vi "Documentation.vi"   [LabVIEW 2019, in "Inst.Transport.lvclass"]
uses:
  Inst.Transport.lvclass
  Typedefs/Inst.Transport.getAll--Cluster.ctl
  Typedefs/Inst.Transport.Configuration--Cluster.ctl
  <userlib>/LevyLab/Instrument Framework/Instrument/Instrument.lvclass
  <vilib>/JKI/JKI SMO/SMO/SMO.lvclass
  <userlib>/LevyLab/Instrument Framework/Instrument UI/Instrument UI.lvclass
  <vilib>/JKI/JKI SMO/SMO.UI/SMO.UI.lvclass
  C:/Program Files (x86)/National Instruments/LabVIEW 2019/user.lib/LevyLab/Instrument Framework/Instrument Types/SCPI/Instrument.SCPI.lvclass
  C:/Program Files (x86)/National Instruments/LabVIEW 2019/user.lib/LevyLab/Instrument Framework/Instrument/Instrument.lvclass
  C:/Program Files (x86)/National Instruments/LabVIEW 2019/vi.lib/JKI/JKI SMO/SMO/SMO.lvclass
  Typedefs/Inst.Transport.PublicCommands--Enum.ctl
  <userlib>/LevyLab/Instrument Framework/Instrument/Typedefs/Instrument.ProtectedCommands--Enum.ctl
  <userlib>/LevyLab/Instrument Framework/Instrument/Typedefs/Instrument.Commands--Enum.ctl
  Typedefs/Inst.Transport.ProtectedCommands--Enum.ctl
  <userlib>/LevyLab/Instrument Framework/Instrument Types/Amplifier/Instrument.Amplifier.lvclass
  <userlib>/LevyLab/Instrument Framework/Instrument Types/CBridge/Instrument.CBridge.lvclass
  <userlib>/LevyLab/Instrument Framework/Instrument Types/Cryostat/Instrument.Cryostat.lvclass
  <userlib>/LevyLab/Instrument Framework/Instrument Types/Delay Line/Instrument.DelayLine.lvclass
  <userlib>/LevyLab/Instrument Framework/Instrument Types/Lockin/Instrument.LockinAPI.lvclass
  <userlib>/LevyLab/Instrument Framework/Instrument Types/Strain/Instrument.Strain.lvclass
  <userlib>/LevyLab/Instrument Framework/Instrument Types/VNA/Instrument.VNA.lvclass
  <userlib>/LevyLab/Instrument Framework/Instrument Types/SCPI/Instrument.SCPI.lvclass
  <userlib>/LevyLab/Instrument Framework/Instrument Types/SignalGenerator/Instrument.SignalGenerator.lvclass
  <userlib>/LevyLab/Instrument Framework/Instrument Types/VSource/Instrument.VSource.lvclass
  d6248588-9140-4ff5-86c8-21cd21a7458c.vi
  7f72b22a-d2f9-4e7f-a221-6a14f9895fe8.vi
  C:/Program Files (x86)/National Instruments/LabVIEW 2019/vi.lib/JKI/JKI SMO/SMO.UI/SMO.UI.lvclass
types:
  T1 = typedef "Inst.Transport.lvclass/Inst.Transport.Configuration--Cluster.ctl" = cluster{"Folder":string, "Comments":string}
  T2 = typedef "Inst.Transport.lvclass/Inst.Transport.getAll--Cluster.ctl" = cluster{"data":variant}
  T3 = typedef "Inst.Transport.lvclass/Inst.Transport.ProtectedCommands--Enum.ctl" = enum16{"setStatus", "showUI", "hideUI"}
  T4 = typedef "Inst.Transport.lvclass/Inst.Transport.PublicCommands--Enum.ctl" = enum16{"startTransport", "stopTransport", "getStatus", "setExptFolder", "setExptComments", "appendExptParam", "clearExptParam", "setExptParam", "setSweepConfig"}
  T5 = typedef "Instrument.lvlib/Instrument.lvclass/Instrument.Commands--Enum.ctl" = enum16{"ACK", "HELP", "IDN", "getAll", "getAllData"}
  T6 = typedef "Instrument.lvlib/Instrument.lvclass/Instrument.ProtectedCommands--Enum.ctl" = enum16{"setConfiguration", "setIDN", "setAll", "setAllData"}
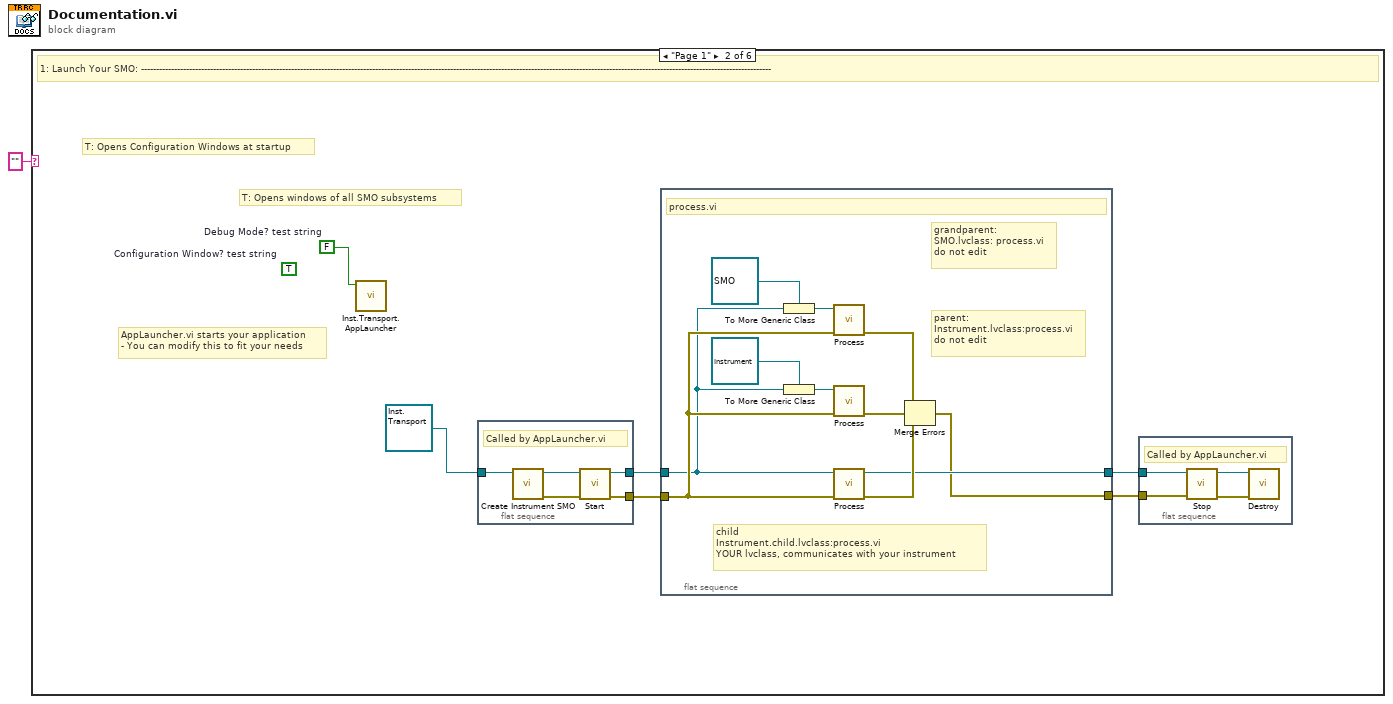
[diagram p0: block diagram]
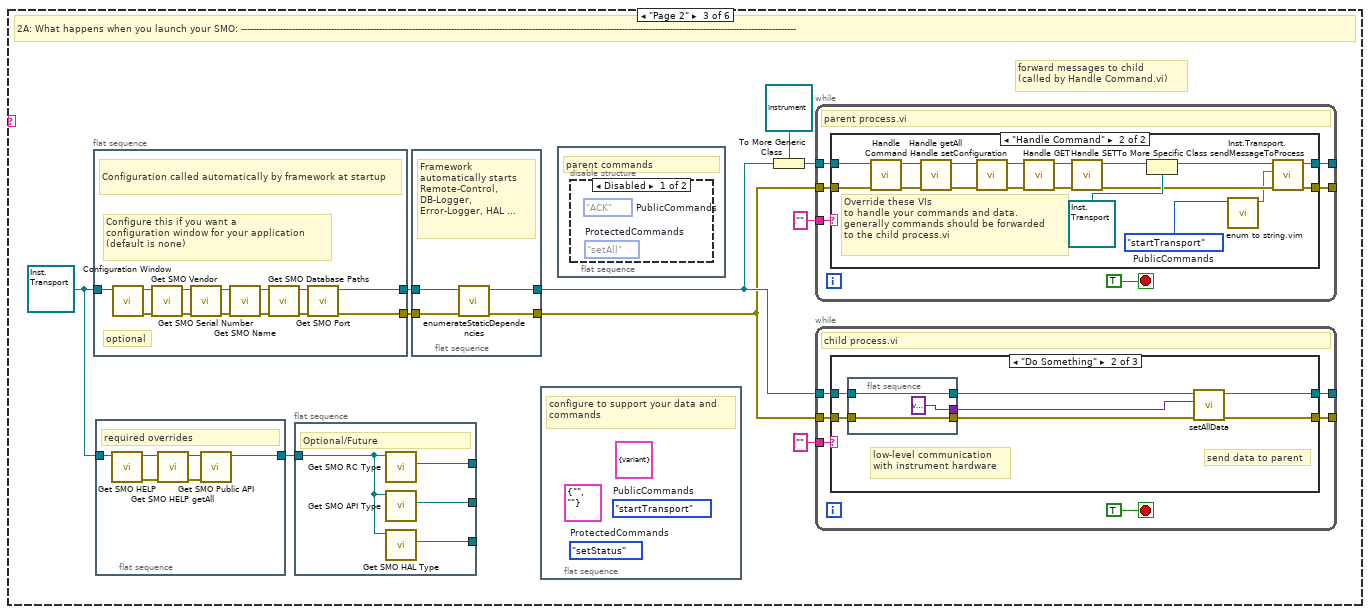
[diagram p3: hidden frame]
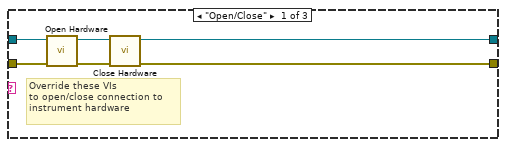
[diagram p5: hidden frame]
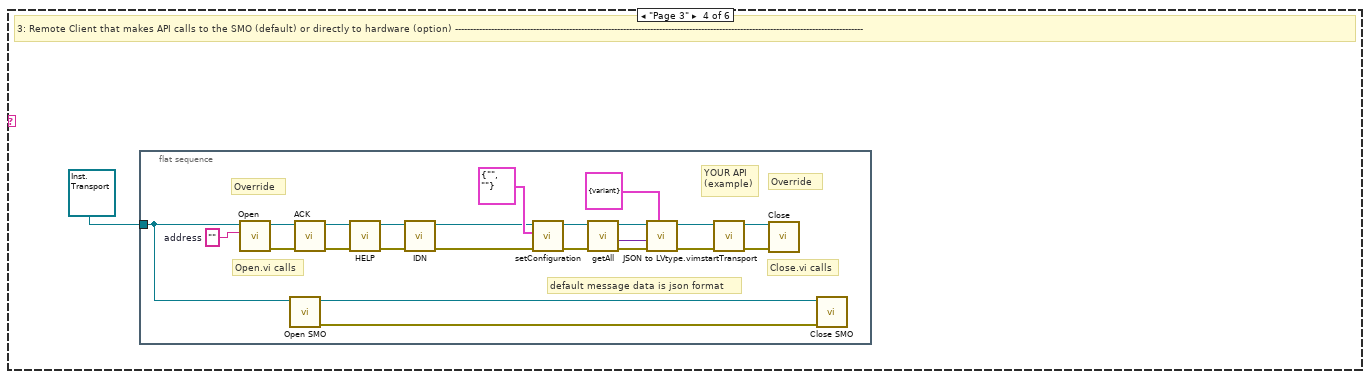
[diagram p8: hidden frame]
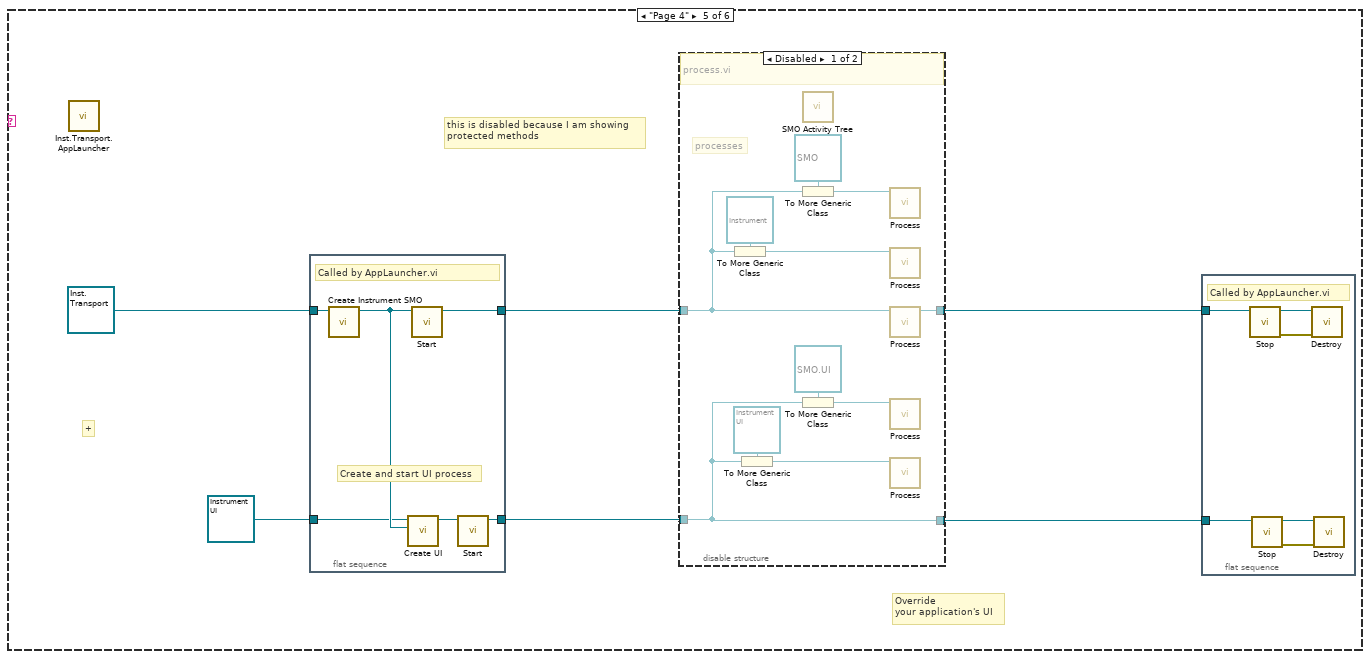
[diagram p9: hidden frame]
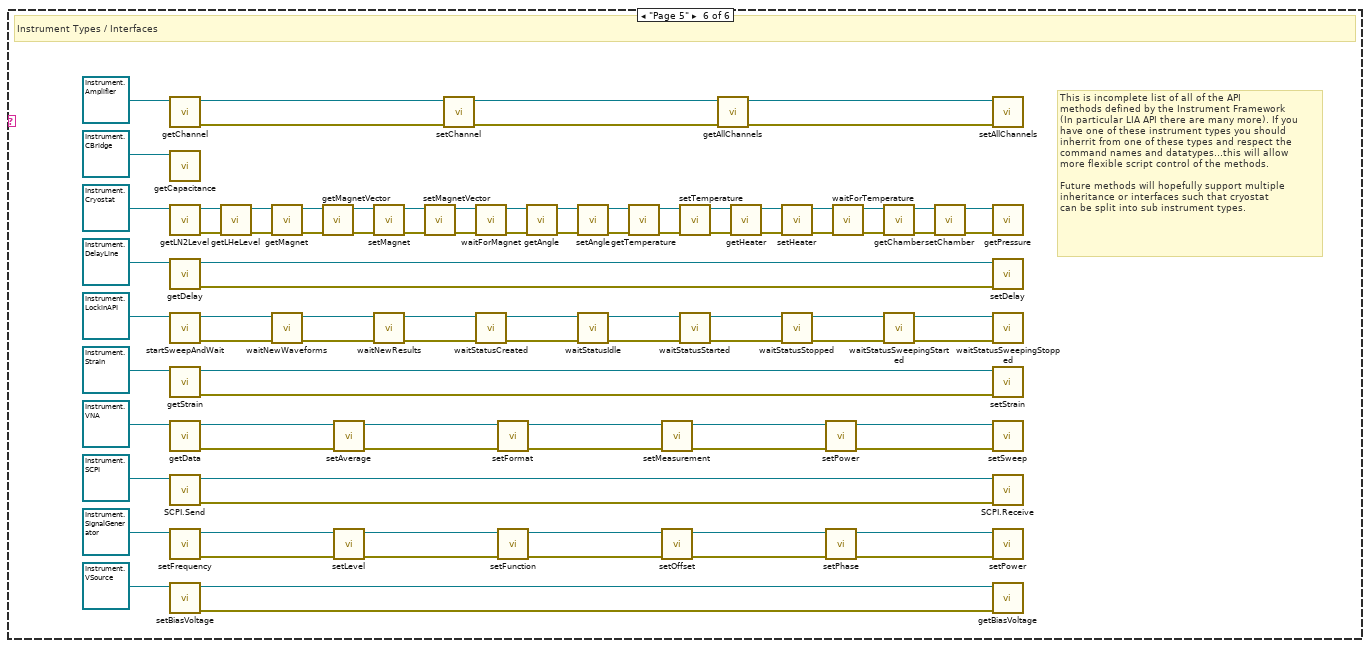
[diagram p11: hidden frame]
diagram:
  n1 = case shown="\"Page 1\"" "" {
    frame Default {
    }
    frame "Page 1" {
      (unwired) TRUE  # Configuration Window? test string
      w7 = FALSE  # Debug Mode? test string
      # "AppLauncher.vi starts your application\n- You can modify this to fit your needs"
      # "T: Opens windows of all SMO subsystems"
      # "T: Opens Configuration Windows at startup"
      # "1: Launch Your SMO: ------------------------------------------------------------------------------------------------------------------------------------------------------------------------------------------------------------------"
      n2 = call "Inst.Transport.AppLauncher.vi"("Debug Mode"=w7) -> ()  [unwired: 10 in, 1 out]
      n3 = flat-sequence {
        tunnel: [w25] -> w3
        tunnel: [w24] -> w5
        tunnel: refnum<class "Inst.Transport.lvclass"> refnum ("Instrument.Template.lvclass") -> [w23]
        frame #0 {
          # "Called by AppLauncher.vi"
          n4 = call <userlib>:"Create Instrument SMO.vi"("Instrument in"=w23) -> ("error out"=w26:errorcluster, "Instrument out"=w27:refnum<class "Inst.Transport.lvclass">)  [unwired: 9 in]
          n5 = call <vilib>:"Start.vi"("error in (no error)"=w26, "SMO"=w27) -> ("error out"=w24:errorcluster, "SMO out"=w25:refnum<class "Inst.Transport.lvclass">)  [unwired: 8 in]
        }
      }
      n6 = flat-sequence {
        tunnel: [w9] -> w6
        tunnel: w5 -> [w17]
        tunnel: [w12] -> w4
        tunnel: w3 -> [w11]
        frame #0 {
          # "child\nInstrument.child.lvclass:process.vi\nYOUR lvclass, communicates with your instrument"
          # "grandparent:\nSMO.lvclass: process.vi\ndo not edit"
          # "parent:\nInstrument.lvclass:process.vi\ndo not edit"
          # "process.vi"
          n7 = To More Generic Class(target class=refnum<class "SMO.lvclass"> refnum ("SMO"), reference=w11) -> (generic class reference=w18:refnum<class "SMO.lvclass">)
          n8 = To More Generic Class(target class=refnum<class "Instrument.lvclass"> refnum ("Instrument"), reference=w11) -> (generic class reference=w16:refnum<class "Instrument.lvclass">)
          n9 = call-dynamic "Process.vi"("error in"=w17, "SMO"=w18) -> ("error out"=w13:errorcluster)  [unwired: 8 in, 1 out]
          n10 = call-dynamic "Process.vi"("error in"=w17, "Instrument"=w16) -> ("error out"=w15:errorcluster)  [unwired: 8 in, 1 out]
          n11 = call-dynamic "Process.vi"("error in"=w17, "Inst.Transport in"=w11) -> ("error out"=w14:errorcluster, "Inst.Transport out"=w12:refnum<class "Inst.Transport.lvclass">)  [unwired: 8 in]
          n12 = Merge Errors(w13, w15, w14) -> (w9:errorcluster)
        }
      }
      n13 = flat-sequence {
        tunnel: w4 -> [w20]
        tunnel: w6 -> [w19]
        frame #0 {
          # "Called by AppLauncher.vi"
          n14 = call <vilib>:"Stop.vi"("error in (no error)"=w19, "SMO"=w20) -> ("error out"=w22:errorcluster, "SMO out"=w21:refnum<class "Inst.Transport.lvclass">)  [unwired: 8 in]
          n15 = call <vilib>:"Destroy.vi"("error in (no error)"=w22, "SMO"=w21) -> ()  [unwired: 9 in, 1 out]
        }
      }
    }
    frame "Page 2" {
      w31 = refnum<class "Inst.Transport.lvclass"> refnum ("Instrument.Template.lvclass")
      # "forward messages to child\n(called by Handle Command.vi)"
      # "2A: What happens when you launch your SMO: -----------------------------------------------------------------------------------------------------------------------------------------------------------------------------------------"
      n16 = flat-sequence {
        tunnel: w31 -> [w58]
        tunnel: [w48] -> w32
        tunnel: [w49] -> w33
        frame #0 {
          # "optional"
          # "Configure this if you want a\nconfiguration window for your application\n(default is none)"
          # "Configuration called automatically by framework at startup"
          n17 = call-dynamic "Configuration Window.vi"("Example Instrument in"=w58) -> ("error out"=w60:errorcluster, "Example Instrument out"=w59:refnum<class "Inst.Transport.lvclass">)  [unwired: 9 in]
          n18 = call-dynamic "Get SMO Vendor.vi"("error in (no error)"=w60, "Inst.Transport in"=w59) -> ("error out"=w50:errorcluster, "Inst.Transport out"=w55:refnum<class "Inst.Transport.lvclass">)  [unwired: 7 in, 1 out]
          n19 = call-dynamic "Get SMO Serial Number.vi"("error in (no error)"=w50, "Inst.Transport in"=w55) -> ("error out"=w51:errorcluster, "Inst.Transport out"=w54:refnum<class "Inst.Transport.lvclass">)  [unwired: 7 in, 1 out]
          n20 = call-dynamic "Get SMO Name.vi"("error in (no error)"=w51, "Inst.Transport in"=w54) -> ("error out"=w52:errorcluster, "Inst.Transport out"=w53:refnum<class "Inst.Transport.lvclass">)  [unwired: 7 in, 1 out]
          n21 = call-dynamic "Get SMO Database Paths.vi"("error in (no error)"=w52, "Inst.Transport in"=w53) -> ("error out"=w56:errorcluster, "Inst.Transport out"=w57:refnum<class "Inst.Transport.lvclass">)  [unwired: 7 in, 1 out]
          n22 = call-dynamic "Get SMO Port.vi"("error in (no error)"=w56, "Inst.Transport in"=w57) -> ("error out"=w48:errorcluster, "Inst.Transport out"=w49:refnum<class "Inst.Transport.lvclass">)  [unwired: 7 in, 1 out]
        }
      }
      n23 = flat-sequence {
        tunnel: w31 -> [w39]
        tunnel: [w38] -> w30
        frame #0 {
          # "required overrides"
          n24 = call-dynamic "Get SMO HELP.vi"("Inst.Transport in"=w39) -> ("error out"=w43:errorcluster, "Inst.Transport out"=w42:refnum<class "Inst.Transport.lvclass">)  [unwired: 8 in, 1 out]
          n25 = call-dynamic "Get SMO HELP getAll.vi"("error in (no error)"=w43, "Inst.Transport in"=w42) -> ("error out"=w40:errorcluster, "Inst.Transport out"=w41:refnum<class "Inst.Transport.lvclass">)  [unwired: 7 in, 1 out]
          n26 = call-dynamic "Get SMO Public API.vi"("error in (no error)"=w40, "Inst.Transport in"=w41) -> ("Inst.Transport out"=w38:refnum<class "Inst.Transport.lvclass">)  [unwired: 7 in, 2 out]
        }
      }
      n27 = flat-sequence {
        tunnel: w30 -> [w64]
        tunnel: [w63] -> _
        tunnel: [w62] -> _
        tunnel: [w61] -> _
        frame #0 {
          # "Optional/Future"
          n28 = call-dynamic "Get SMO RC Type.vi"("Instrument in"=w64) -> ("RemoteControl"=w63:refnum<class "RemoteControl.lvclass">)  [unwired: 8 in, 2 out]
          n29 = call-dynamic "Get SMO API Type.vi"("Instrument in"=w64) -> ("API"=w62:refnum<class "API.lvclass">)  [unwired: 8 in, 2 out]
          n30 = call-dynamic "Get SMO HAL Type.vi"("Instrument in"=w64) -> ("Dependencies.HAL"=w61:refnum<class "HAL.lvclass">)  [unwired: 8 in, 2 out]
        }
      }
      n31 = flat-sequence {
        tunnel: w33 -> [w47]
        tunnel: w32 -> [w46]
        tunnel: [w45] -> w29
        tunnel: [w44] -> w28
        frame #0 {
          # "Framework automatically starts\nRemote-Control, DB-Logger, Error-Logger, HAL ..."
          n32 = call-dynamic "enumerateStaticDependencies.vi"("error in (no error)"=w46, "Instrument"=w47) -> ("error out"=w44:errorcluster, "Instrument out"=w45:refnum<class "Inst.Transport.lvclass">)  [unwired: 7 in, 1 out]
        }
      }
      n33 = flat-sequence {
        frame #0 {
          (unwired) Inst.Transport.ProtectedCommands--Enum."setStatus"  # ProtectedCommands
          (unwired) T1 {"Folder"="", "Comments"=""} ("Configuration")
          (unwired) T2 {"data"=variant(string "")} ("getAll")
          (unwired) Inst.Transport.PublicCommands--Enum."startTransport"  # PublicCommands
          # "configure to support your data and commands"
        }
      }
      n34 = flat-sequence {
        frame #0 {
          # "parent commands"
          n35 = disable-structure shown="Disabled" {
            frame Disabled {
              (unwired) Instrument.Commands--Enum."ACK"  # PublicCommands
              (unwired) Instrument.ProtectedCommands--Enum."setAll"  # ProtectedCommands
            }
            frame Enabled {
            }
          }
        }
      }
      n36 = To More Generic Class(target class=refnum<class "Instrument.lvclass"> refnum ("Instrument"), reference=w29) -> (generic class reference=w34:refnum<class "Instrument.lvclass">)
      n37 = while {
        tunnel: "" -> [w94]
        tunnel: w34 -> [w92]
        tunnel: [w91] -> _
        tunnel: w28 -> [w90]
        tunnel: [w89] -> _
        stop <- TRUE stop-if-true
        # "parent process.vi"
        n38 = case shown="\"Handle Command\"" w94 {
          tunnel: w92 -> [w96 w114]
          tunnel: [w96 w108] -> w91
          tunnel: w90 -> [w95 w113]
          tunnel: [w95 w107] -> w89
          frame Default {
          }
          frame "Handle Command" {
            w98 = Inst.Transport.PublicCommands--Enum."startTransport"  # PublicCommands
            # "Override these VIs\nto handle your commands and data.\ngenerally commands should be forwarded\nto the child process.vi"
            n39 = call-dynamic "Handle Command.vi"("error in (no error)"=w113, "Instrument in"=w114) -> ("error out"=w109:errorcluster, "Instrument out"=w112:refnum<class "Instrument.lvclass">)  [unwired: 6 in, 2 out]
            n40 = call-dynamic "Handle getAll.vi"("error in (no error)"=w109, "Instrument in"=w112) -> ("error out"=w110:errorcluster, "Instrument out"=w111:refnum<class "Instrument.lvclass">)  [unwired: 7 in, 1 out]
            n41 = call-dynamic "Handle setConfiguration.vi"("error in (no error)"=w110, "Instrument in"=w111) -> ("error out"=w103:errorcluster, "Instrument out"=w104:refnum<class "Instrument.lvclass">)  [unwired: 8 in]
            n42 = call-dynamic "Handle GET.vi"("error in (no error)"=w103, "Instrument in"=w104) -> ("error out"=w101:errorcluster, "Instrument out"=w102:refnum<class "Instrument.lvclass">)  [unwired: 7 in, 1 out]
            n43 = call-dynamic "Handle SET.vi"("error in (no error)"=w101, "Instrument in"=w102) -> ("error out"=w99:errorcluster, "Instrument out"=w100:refnum<class "Instrument.lvclass">)  [unwired: 7 in, 1 out]
            n44 = To More Specific Class(target class=refnum<class "Inst.Transport.lvclass"> refnum ("Instrument.Template.lvclass"), reference=w100) -> (specific class reference=w106:refnum<class "Inst.Transport.lvclass">)  [unwired: 1 in, 1 out]
            n45 = call "enum to string.vim"("enum in"=w98) -> ("string out"=w97:string)  [unwired: 9 in, 1 out]
            n46 = call "Inst.Transport.sendMessageToProcess.vi"("error in (no error)"=w99, "Command"=w97, "Inst.Transport in"=w106) -> ("error out"=w107:errorcluster, "Inst.Transport out"=w108:refnum<class "Inst.Transport.lvclass">)  [unwired: 7 in]
          }
        }
      }
      n47 = while {
        tunnel: "" -> [w70]
        tunnel: w29 -> [w68]
        tunnel: [w67] -> _
        tunnel: w28 -> [w66]
        tunnel: [w65] -> _
        stop <- TRUE stop-if-true
        # "child process.vi"
        n48 = case shown="\"Do Something\"" w70 {
          tunnel: w68 -> [w73 w82 w88]
          tunnel: [w72 w79 w88] -> w67
          tunnel: w66 -> [w76 w83 w87]
          tunnel: [w71 w78 w87] -> w65
          frame "Open/Close" {
            # "Override these VIs\nto open/close connection to\ninstrument hardware"
            n49 = call-dynamic "Open Hardware.vi"("error in (no error)"=w76, "Instrument in"=w73) -> ("error out"=w75:errorcluster, "Instrument out"=w74:refnum<class "Inst.Transport.lvclass">)  [unwired: 8 in]
            n50 = call-dynamic "Close Hardware.vi"("error in (no error)"=w75, "Instrument in"=w74) -> ("error out"=w71:errorcluster, "Instrument out"=w72:refnum<class "Inst.Transport.lvclass">)  [unwired: 8 in]
          }
          frame "Do Something" {
            # "low-level communication\nwith instrument hardware"
            # "send data to parent"
            n51 = flat-sequence {
              tunnel: w83 -> [w86]
              tunnel: [w86] -> w77
              tunnel: w82 -> [w85]
              tunnel: [w85] -> w80
              tunnel: [variant ("Data")] -> w81
              frame #0 {
              }
            }
            n52 = call <userlib>:"setAllData.vi"("error in (no error)"=w77, "AllData"=w81, "Instrument in"=w80) -> ("error out"=w78:errorcluster, "Instrument out"=w79:refnum<class "Inst.Transport.lvclass">)  [unwired: 7 in]
          }
          frame Default {
          }
        }
      }
    }
    frame "Page 3" {
      # "3: Remote Client that makes API calls to the SMO (default) or directly to hardware (option) ----------------------------------------------------------------------------------------------------------------------------------------"
      n53 = flat-sequence {
        tunnel: refnum<class "Inst.Transport.lvclass"> refnum ("Instrument.Template.lvclass") -> [w125]
        frame #0 {
          w128 = ""  # address
          # "default message data is json format"
          # "Close.vi calls"
          # "Open.vi calls"
          # "YOUR API\n(example)"
          # "Override"
          # "Override"
          n54 = call-dynamic "Open.vi"("address"=w128, "Inst.Transport in"=w125) -> ("error out"=w137:errorcluster, "Inst.Transport out"=w136:refnum<class "Inst.Transport.lvclass">)  [unwired: 8 in]
          n55 = call <userlib>:"Open SMO.vi"("Instrument in"=w125) -> ("error out"=w126:errorcluster, "Instrument out"=w127:refnum<class "Inst.Transport.lvclass">)  [unwired: 9 in]
          n56 = call <userlib>:"ACK.vi"("error in (no error)"=w137, "Instrument in"=w136) -> ("error out"=w135:errorcluster, "Instrument out"=w134:refnum<class "Inst.Transport.lvclass">)  [unwired: 7 in, 1 out]
          n57 = call <userlib>:"HELP.vi"("error in (no error)"=w135, "Instrument in"=w134) -> ("error out"=w118:errorcluster, "Instrument in"=w119:refnum<class "Inst.Transport.lvclass">)  [unwired: 7 in, 1 out]
          n58 = call <userlib>:"IDN.vi"("error in (no error)"=w118, "Instrument in"=w119) -> ("error out"=w116:errorcluster, "Instrument in"=w117:refnum<class "Inst.Transport.lvclass">)  [unwired: 7 in, 1 out]
          n59 = call <userlib>:"setConfiguration.vi"("error in (no error)"=w116, "Configuration"=T1 {"Folder"="", "Comments"=""}, "Instrument in"=w117) -> ("error out"=w129:errorcluster, "Instrument out"=w130:refnum<class "Inst.Transport.lvclass">)  [unwired: 7 in]
          n60 = call <userlib>:"getAll.vi"("error in (no error)"=w129, "Instrument in"=w130) -> ("error out"=w124:errorcluster, "getAll"=w120:variant, "Instrument out"=w121:refnum<class "Inst.Transport.lvclass">)  [unwired: 7 in]
          n61 = call "JSON to LVtype.vim"("type"=T2 {"data"=variant(string "")} ("getAll"), "error in (no error)"=w124, "JSON Data in"=w120) -> ("error out"=w122:errorcluster)  [unwired: 7 in, 1 out]
          n62 = call "startTransport.vi"("error in (no error)"=w122, "Inst.Transport in"=w121) -> ("error out"=w132:errorcluster, "Inst.Transport out"=w133:refnum<class "Inst.Transport.lvclass">)  [unwired: 8 in]
          n63 = call-dynamic "Close.vi"("error in (no error)"=w132, "Inst.Transport in"=w133) -> ()  [unwired: 8 in, 2 out]
          n64 = call <userlib>:"Close SMO.vi"("error in (no error)"=w126, "Instrument in"=w127) -> ()  [unwired: 8 in, 2 out]
        }
      }
    }
    frame "Page 4" {
      # "this is disabled because I am showing\nprotected methods"
      # "Override\nyour application's UI"
      # "+"
      n65 = call "Inst.Transport.AppLauncher.vi"() -> ()  [unwired: 11 in, 1 out]
      n66 = flat-sequence {
        tunnel: [w155] -> w141
        tunnel: refnum<class "Inst.Transport.lvclass"> refnum ("Instrument.Template.lvclass") -> [w154]
        tunnel: refnum<class "Instrument UI.lvclass"> refnum ("Instrument UI") -> [w152]
        tunnel: [w150] -> w140
        frame #0 {
          # "Create and start UI process"
          # "Called by AppLauncher.vi"
          n67 = call <userlib>:"Create Instrument SMO.vi"("Instrument in"=w154) -> ("Instrument out"=w153:refnum<class "Inst.Transport.lvclass">)  [unwired: 9 in, 1 out]
          n68 = call <userlib>:"Create UI.vi"("Instrument in"=w153, "Instrument UI"=w152) -> ("Instrument UI out"=w151:refnum<class "Instrument UI.lvclass">)  [unwired: 8 in, 1 out]
          n69 = call <vilib>:"Start.vi"("SMO"=w153) -> ("SMO out"=w155:refnum<class "Inst.Transport.lvclass">)  [unwired: 9 in, 1 out]
          n70 = call <vilib>:"Start.vi"("SMO"=w151) -> ("SMO out"=w150:refnum<class "Instrument UI.lvclass">)  [unwired: 9 in, 1 out]
        }
      }
      n71 = disable-structure shown="Disabled" {
        disable-tunnel: [w166 w168] -> w142
        disable-tunnel: w141 -> [w165 w168]
        disable-tunnel: w140 -> [w156 w167]
        disable-tunnel: [w156 w167] -> w139
        frame Disabled {
          # "processes"
          # "process.vi"
          n72 = To More Generic Class(target class=refnum<class "Instrument.lvclass"> refnum ("Instrument"), reference=w165) -> (generic class reference=w163:refnum<class "Instrument.lvclass">)
          n73 = To More Generic Class(target class=refnum<class "Instrument UI.lvclass"> refnum ("Instrument UI"), reference=w156) -> (generic class reference=w159:refnum<class "Instrument UI.lvclass">)
          n74 = call <vilib>:"SMO Activity Tree.vi"() -> ()  [unwired: 12 in]
          n75 = To More Generic Class(target class=refnum<class "SMO.lvclass"> refnum ("SMO"), reference=w165) -> (generic class reference=w164:refnum<class "SMO.lvclass">)
          n76 = To More Generic Class(target class=refnum<class "SMO.UI.lvclass"> refnum ("SMO.UI"), reference=w156) -> (generic class reference=w157:refnum<class "SMO.UI.lvclass">)
          n77 = call-dynamic "Process.vi"("SMO"=w164) -> ()  [unwired: 9 in, 2 out]
          n78 = call-dynamic "Process.vi"("Instrument"=w163) -> ()  [unwired: 9 in, 2 out]
          n79 = call-dynamic "Process.vi"("Inst.Transport in"=w165) -> ("Inst.Transport out"=w166:refnum<class "Inst.Transport.lvclass">)  [unwired: 9 in, 1 out]
          n80 = call-dynamic "Process.vi"("SMO.UI"=w157) -> ()  [unwired: 9 in, 2 out]
          n81 = call-dynamic "Process.vi"("Instrument UI in"=w159) -> ()  [unwired: 9 in, 2 out]
        }
        frame Enabled {
        }
      }
      n82 = flat-sequence {
        tunnel: w142 -> [w147]
        tunnel: w139 -> [w145]
        frame #0 {
          # "Called by AppLauncher.vi"
          n83 = call <vilib>:"Stop.vi"("SMO"=w147) -> ("error out"=w149:errorcluster, "SMO out"=w148:refnum<class "Inst.Transport.lvclass">)  [unwired: 9 in]
          n84 = call <vilib>:"Stop.vi"("SMO"=w145) -> ("error out"=w146:errorcluster, "SMO out"=w144:refnum<class "Instrument UI.lvclass">)  [unwired: 9 in]
          n85 = call <vilib>:"Destroy.vi"("error in (no error)"=w149, "SMO"=w148) -> ()  [unwired: 9 in, 1 out]
          n86 = call <vilib>:"Destroy.vi"("error in (no error)"=w146, "SMO"=w144) -> ()  [unwired: 9 in, 1 out]
        }
      }
    }
    frame "Page 5" {
      # "This is incomplete list of all of the API\nmethods defined by the Instrument Framework\n(In particular LIA API there are many more). If you\nhave one of these instrument types you should\ninherrit from one of these types and respect the \ncommand names and datatypes...this will allow\nmore flexible script control of the methods.\n\nFuture methods will hopefully support multiple\ninheritance or interfaces such that cryostat\ncan be split into sub instrument types."
      # "Instrument Types / Interfaces"
      n87 = call-dynamic "getChannel.vi"("Instrument.Amplifier in"=refnum<class "Instrument.Amplifier.lvclass"> refnum ("Instrument.Amplifier.lvclass")) -> ("error out"=w249:errorcluster, "Instrument.Amplifier out"=w250:refnum<class "Instrument.Amplifier.lvclass">)  [unwired: 8 in, 1 out]
      n88 = call-dynamic "getCapacitance.vi"("Instrument.CBridge in"=refnum<class "Instrument.CBridge.lvclass"> refnum ("Instrument.CBridge.lvclass")) -> ()  [unwired: 8 in, 3 out]
      n89 = call-dynamic "getLN2Level.vi"("Instrument.Cryostat in"=refnum<class "Instrument.Cryostat.lvclass"> refnum ("Instrument.Cryostat.lvclass")) -> ("error out"=w243:errorcluster, "Instrument.Cryostat out"=w244:refnum<class "Instrument.Cryostat.lvclass">)  [unwired: 8 in, 1 out]
      n90 = call <userlib>:"getDelay.vi"("Instrument.DelayLine in"=refnum<class "Instrument.DelayLine.lvclass"> refnum ("Instrument.DelayLine.lvclass")) -> ("error out"=w211:errorcluster, "Instrument.DelayLine out"=w212:refnum<class "Instrument.DelayLine.lvclass">)  [unwired: 7 in, 2 out]
      n91 = call-dynamic "startSweepAndWait.vi"("Instrument.LockinAPI in"=refnum<class "Instrument.LockinAPI.lvclass"> refnum ("Instrument.LockinAPI.lvclass")) -> ("error out"=w209:errorcluster, "Instrument.LockinAPI out"=w210:refnum<class "Instrument.LockinAPI.lvclass">)  [unwired: 9 in]
      n92 = call-dynamic "getStrain.vi"("Instrument.Strain in"=refnum<class "Instrument.Strain.lvclass"> refnum ("Instrument.Strain.lvclass")) -> ("error out"=w193:errorcluster, "Instrument.Strain out"=w194:refnum<class "Instrument.Strain.lvclass">)  [unwired: 8 in, 1 out]
      n93 = call-dynamic "getData.vi"("Instrument.VSource in"=refnum<class "Instrument.VNA.lvclass"> refnum ("Instrument.VNA.lvclass")) -> ("error out"=w191:errorcluster, "Instrument.VSource out"=w192:refnum<class "Instrument.VNA.lvclass">)  [unwired: 8 in, 1 out]
      n94 = call-dynamic "SCPI.Send.vi"("Instrument.SCPI in"=refnum<class "Instrument.SCPI.lvclass"> refnum ("Instrument.SCPI.lvclass")) -> ("error out"=w181:errorcluster, "Instrument.SCPI out"=w182:refnum<class "Instrument.SCPI.lvclass">)  [unwired: 9 in]
      n95 = call-dynamic "setFrequency.vi"("Instrument.SignalGenerator in"=refnum<class "Instrument.SignalGenerator.lvclass"> refnum ("Instrument.SignalGenerator.lvclass")) -> ("error out"=w179:errorcluster, "Instrument.SignalGenerator out"=w180:refnum<class "Instrument.SignalGenerator.lvclass">)  [unwired: 9 in]
      n96 = call-dynamic "setBiasVoltage.vi"("Instrument.VSource in"=refnum<class "Instrument.VSource.lvclass"> refnum ("Instrument.VSource.lvclass")) -> ("error out"=w169:errorcluster, "Instrument.VSource out"=w170:refnum<class "Instrument.VSource.lvclass">)  [unwired: 9 in]
      n97 = call-dynamic "getLHeLevel.vi"("error in (no error)"=w243, "Instrument.Cryostat in"=w244) -> ("error out"=w241:errorcluster, "Instrument.Cryostat out"=w242:refnum<class "Instrument.Cryostat.lvclass">)  [unwired: 7 in, 1 out]
      n98 = call-dynamic "getMagnet.vi"("error in (no error)"=w241, "Instrument.Cryostat in"=w242) -> ("error out"=w239:errorcluster, "Instrument.Cryostat out"=w240:refnum<class "Instrument.Cryostat.lvclass">)  [unwired: 5 in, 3 out]
      n99 = call-dynamic "waitNewWaveforms.vi"("error in (no error)"=w209, "Instrument.LockinAPI in"=w210) -> ("error out"=w207:errorcluster, "Instrument.LockinAPI out"=w208:refnum<class "Instrument.LockinAPI.lvclass">)  [unwired: 7 in, 1 out]
      n100 = call-dynamic "getMagnetVector.vi"("error in (no error)"=w239, "Instrument.Cryostat in"=w240) -> ("error out"=w237:errorcluster, "Instrument.Cryostat out"=w238:refnum<class "Instrument.Cryostat.lvclass">)  [unwired: 5 in, 3 out]
      n101 = call-dynamic "setAverage.vi"("error in (no error)"=w191, "Instrument.VSource in"=w192) -> ("error out"=w189:errorcluster, "Instrument.VSource out"=w190:refnum<class "Instrument.VNA.lvclass">)  [unwired: 8 in]
      n102 = call-dynamic "setLevel.vi"("error in (no error)"=w179, "Instrument.SignalGenerator in"=w180) -> ("error out"=w177:errorcluster, "Instrument.SignalGenerator out"=w178:refnum<class "Instrument.SignalGenerator.lvclass">)  [unwired: 8 in]
      n103 = call-dynamic "setMagnet.vi"("error in (no error)"=w237, "Instrument.Cryostat in"=w238) -> ("error out"=w235:errorcluster, "Instrument.Cryostat out"=w236:refnum<class "Instrument.Cryostat.lvclass">)  [unwired: 8 in]
      n104 = call-dynamic "waitNewResults.vi"("error in (no error)"=w207, "Instrument.LockinAPI in"=w208) -> ("error out"=w205:errorcluster, "Instrument.LockinAPI out"=w206:refnum<class "Instrument.LockinAPI.lvclass">)  [unwired: 7 in, 1 out]
      n105 = call-dynamic "setMagnetVector.vi"("error in (no error)"=w235, "Instrument.Cryostat in"=w236) -> ("error out"=w233:errorcluster, "Instrument.Cryostat out"=w234:refnum<class "Instrument.Cryostat.lvclass">)  [unwired: 8 in]
      n106 = call-dynamic "setChannel.vi"("error in (no error)"=w249, "Instrument.Amplifier in"=w250) -> ("error out"=w247:errorcluster, "Instrument.Amplifier out"=w248:refnum<class "Instrument.Amplifier.lvclass">)  [unwired: 8 in]
      n107 = call <userlib>:"waitForMagnet.vi"("error in (no error)"=w233, "Instrument.Cryostat in"=w234) -> ("error out"=w231:errorcluster, "Instrument.Cryostat out"=w232:refnum<class "Instrument.Cryostat.lvclass">)  [unwired: 8 in]
      n108 = call-dynamic "waitStatusCreated.vi"("error in (no error)"=w205, "Instrument.LockinAPI in"=w206) -> ("error out"=w203:errorcluster, "Instrument.LockinAPI out"=w204:refnum<class "Instrument.LockinAPI.lvclass">)  [unwired: 8 in]
      n109 = call-dynamic "setFormat.vi"("error in (no error)"=w189, "Instrument.VSource in"=w190) -> ("error out"=w187:errorcluster, "Instrument.VSource out"=w188:refnum<class "Instrument.VNA.lvclass">)  [unwired: 8 in]
      n110 = call-dynamic "setFunction.vi"("error in (no error)"=w177, "Instrument.SignalGenerator in"=w178) -> ("error out"=w175:errorcluster, "Instrument.SignalGenerator out"=w176:refnum<class "Instrument.SignalGenerator.lvclass">)  [unwired: 8 in]
      n111 = call-dynamic "getAngle.vi"("error in (no error)"=w231, "Instrument.Cryostat in"=w232) -> ("error out"=w229:errorcluster, "Instrument.Cryostat out"=w230:refnum<class "Instrument.Cryostat.lvclass">)  [unwired: 5 in, 3 out]
      n112 = call-dynamic "setAngle.vi"("error in (no error)"=w229, "Instrument.Cryostat in"=w230) -> ("error out"=w227:errorcluster, "Instrument.Cryostat out"=w228:refnum<class "Instrument.Cryostat.lvclass">)  [unwired: 8 in]
      n113 = call-dynamic "waitStatusIdle.vi"("error in (no error)"=w203, "Instrument.LockinAPI in"=w204) -> ("error out"=w201:errorcluster, "Instrument.LockinAPI out"=w202:refnum<class "Instrument.LockinAPI.lvclass">)  [unwired: 8 in]
      n114 = call-dynamic "getTemperature.vi"("error in (no error)"=w227, "Instrument.Cryostat in"=w228) -> ("error out"=w225:errorcluster, "Instrument.Cryostat out"=w226:refnum<class "Instrument.Cryostat.lvclass">)  [unwired: 5 in, 3 out]
      n115 = call-dynamic "setMeasurement.vi"("error in (no error)"=w187, "Instrument.VSource in"=w188) -> ("error out"=w185:errorcluster, "Instrument.VSource out"=w186:refnum<class "Instrument.VNA.lvclass">)  [unwired: 8 in]
      n116 = call-dynamic "setOffset.vi"("error in (no error)"=w175, "Instrument.SignalGenerator in"=w176) -> ("error out"=w173:errorcluster, "Instrument.SignalGenerator out"=w174:refnum<class "Instrument.SignalGenerator.lvclass">)  [unwired: 8 in]
      n117 = call-dynamic "setTemperature.vi"("error in (no error)"=w225, "Instrument.Cryostat in"=w226) -> ("error out"=w223:errorcluster, "Instrument.Cryostat out"=w224:refnum<class "Instrument.Cryostat.lvclass">)  [unwired: 8 in]
      n118 = call-dynamic "waitStatusStarted.vi"("error in (no error)"=w201, "Instrument.LockinAPI in"=w202) -> ("error out"=w199:errorcluster, "Instrument.LockinAPI out"=w200:refnum<class "Instrument.LockinAPI.lvclass">)  [unwired: 8 in]
      n119 = call-dynamic "getAllChannels.vi"("error in (no error)"=w247, "Instrument.Amplifier in"=w248) -> ("error out"=w245:errorcluster, "Instrument.Amplifier out"=w246:refnum<class "Instrument.Amplifier.lvclass">)  [unwired: 7 in, 1 out]
      n120 = call-dynamic "getHeater.vi"("error in (no error)"=w223, "Instrument.Cryostat in"=w224) -> ("error out"=w221:errorcluster, "Instrument.Cryostat out"=w222:refnum<class "Instrument.Cryostat.lvclass">)  [unwired: 6 in, 2 out]
      n121 = call-dynamic "setHeater.vi"("error in (no error)"=w221, "Instrument.Cryostat in"=w222) -> ("error out"=w219:errorcluster, "Instrument.Cryostat out"=w220:refnum<class "Instrument.Cryostat.lvclass">)  [unwired: 8 in]
      n122 = call-dynamic "waitStatusStopped.vi"("error in (no error)"=w199, "Instrument.LockinAPI in"=w200) -> ("error out"=w197:errorcluster, "Instrument.LockinAPI out"=w198:refnum<class "Instrument.LockinAPI.lvclass">)  [unwired: 8 in]
      n123 = call-dynamic "setPower.vi"("error in (no error)"=w185, "Instrument.VSource in"=w186) -> ("error out"=w183:errorcluster, "Instrument.VSource out"=w184:refnum<class "Instrument.VNA.lvclass">)  [unwired: 8 in]
      n124 = call-dynamic "setPhase.vi"("error in (no error)"=w173, "Instrument.SignalGenerator in"=w174) -> ("error out"=w171:errorcluster, "Instrument.SignalGenerator out"=w172:refnum<class "Instrument.SignalGenerator.lvclass">)  [unwired: 8 in]
      n125 = call <userlib>:"waitForTemperature.vi"("error in (no error)"=w219, "Instrument.Cryostat in"=w220) -> ("error out"=w217:errorcluster, "Instrument.Cryostat out"=w218:refnum<class "Instrument.Cryostat.lvclass">)  [unwired: 8 in]
      n126 = call-dynamic "getChamber.vi"("error in (no error)"=w217, "Instrument.Cryostat in"=w218) -> ("error out"=w215:errorcluster, "Instrument.Cryostat out"=w216:refnum<class "Instrument.Cryostat.lvclass">)  [unwired: 7 in, 1 out]
      n127 = call-dynamic "waitStatusSweepingStarted.vi"("error in (no error)"=w197, "Instrument.LockinAPI in"=w198) -> ("error out"=w195:errorcluster, "Instrument.LockinAPI out"=w196:refnum<class "Instrument.LockinAPI.lvclass">)  [unwired: 8 in]
      n128 = call-dynamic "setChamber.vi"("error in (no error)"=w215, "Instrument.Cryostat in"=w216) -> ("error out"=w213:errorcluster, "Instrument.Cryostat out"=w214:refnum<class "Instrument.Cryostat.lvclass">)  [unwired: 8 in]
      n129 = call-dynamic "setAllChannels.vi"("error in (no error)"=w245, "Instrument.Amplifier in"=w246) -> ()  [unwired: 8 in, 2 out]
      n130 = call-dynamic "getPressure.vi"("error in (no error)"=w213, "Instrument.Cryostat in"=w214) -> ()  [unwired: 6 in, 4 out]
      n131 = call-dynamic "setDelay.vi"("error in (no error)"=w211, "Instrument.Delay in"=w212) -> ()  [unwired: 8 in, 2 out]
      n132 = call-dynamic "waitStatusSweepingStopped.vi"("error in (no error)"=w195, "Instrument.LockinAPI in"=w196) -> ()  [unwired: 8 in, 2 out]
      n133 = call-dynamic "setStrain.vi"("error in (no error)"=w193, "Instrument.Strain in"=w194) -> ()  [unwired: 8 in, 2 out]
      n134 = call-dynamic "setSweep.vi"("error in (no error)"=w183, "Instrument.VSource in"=w184) -> ()  [unwired: 8 in, 2 out]
      n135 = call-dynamic "SCPI.Receive.vi"("error in (no error)"=w181, "Instrument.SCPI in"=w182) -> ()  [unwired: 7 in, 3 out]
      n136 = call-dynamic "setPower.vi"("error in (no error)"=w171, "Instrument.SignalGenerator in"=w172) -> ()  [unwired: 8 in, 2 out]
      n137 = call-dynamic "getBiasVoltage.vi"("error in (no error)"=w169, "Instrument.VSource in"=w170) -> ()  [unwired: 7 in, 3 out]
    }
  }
